vi "Stable.vi"(8 "Pulse Width (sec)":dbl(knob)=0.5044674819294696 scale=0.0..1.0, 11 "Signal Input":bool) -> (0 "Stable":bool)   [LabVIEW 2011]
panel:
  out "Start":bool
  out "Ref Time Stamp":timestamp
  out "Ready":bool
  out "RPM Control Response":cluster{i16, i16}(graph)
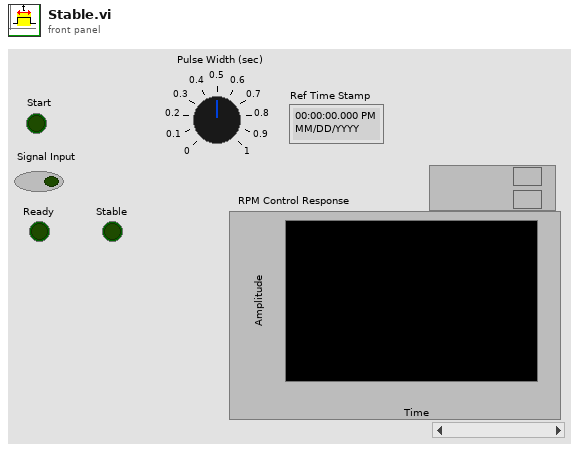
[diagram p1: front panel]
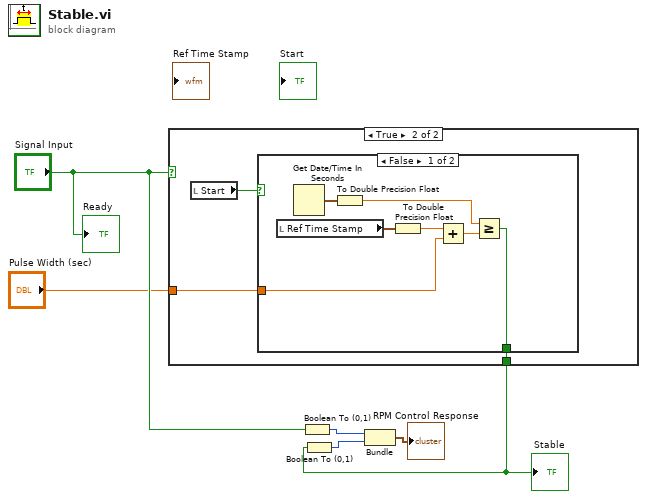
[diagram p0: block diagram]
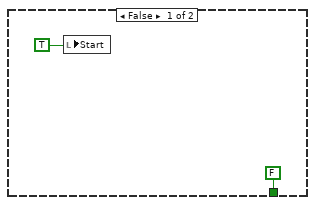
[diagram p2: hidden frame]
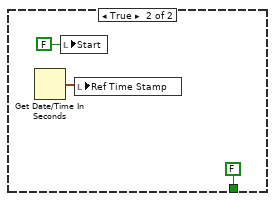
[diagram p3: hidden frame]
diagram:
  n1 = case shown="True" "Signal Input" {
    tunnel: [FALSE w10] -> w3
    tunnel: "Pulse Width (sec)" -> [_ w9]
    frame False {
      n2 = local write "Start"(TRUE) -> ()
    }
    frame True {
      n3 = local read "Start"() -> (w11:bool)
      n4 = case shown="False" w11 {
        tunnel: [w13 FALSE] -> w10
        tunnel: w9 -> [w12 _]
        frame False {
          n5 = local read "Ref Time Stamp"() -> (w17:timestamp)
          n6 = Get Date/Time In Seconds() -> (seconds since 1Jan1904=w18:timestamp)
          n7 = To Double Precision Float(number=w18) -> (double precision float=w14:dbl)
          n8 = To Double Precision Float(number=w17) -> (double precision float=w16:dbl)
          n9 = Add(x=w16, y=w12) -> (x+y=w15:dbl)
          n10 = Greater Or Equal?(x=w14, y=w15) -> (x >= y?=w13:bool)
        }
        frame True {
          n11 = Get Date/Time In Seconds() -> (seconds since 1Jan1904=w21:timestamp)
          n12 = local write "Start"(FALSE ("Start")) -> ()
          n13 = local write "Ref Time Stamp"(w21) -> ()
        }
      }
    }
  }
  "Stable" <- w3
  n14 = Boolean To (0,1)(Boolean="Signal Input") -> (0, 1=w6:i16)
  n15 = Boolean To (0,1)(Boolean=w3) -> (0, 1=w5:i16)
  n16 = Bundle(w6, w5) -> (→"RPM Control Response":cluster{i16, i16})  [unwired: 1 out]
  "Ready" <- "Signal Input"
